vi "Fetch Measurement (Fast Read).vi"(8 "error in (no error)":errorcluster, 10 "Timeout (10000 ms)":u32=10000, 11 "VISA resource name":refnum<visa-resource-name>) -> (0 "error out":errorcluster, 1 "End of Data?":bool, 2 "Measurements":dbl[](array[numeric]) format="%#_24g", 3 "VISA resource name out":refnum<visa-resource-name>)   [LabVIEW 2014, in "Agilent 34401.lvlib"]
doc: "Fetches measurement from the instrument. This VI sends the \"R?\" command to the instrument and is to be used after \"FORM:DATA REAL,64;:FORM:BORD NORM;:INIT;\" has been called. The VI will retrieve and delete the existent data from the instrument's internal buffer. This VI should be called repeatedly until End of Data? is True.\n\n<B>Note:</B>\n\nThis VI is called by <B>Fetch Measurement VI</B> in the following cases:\n(1) Model = 34410/34411 and Math = Off"
uses:
  <instrlib>/Agilent 34401/Agilent 34401.lvlib
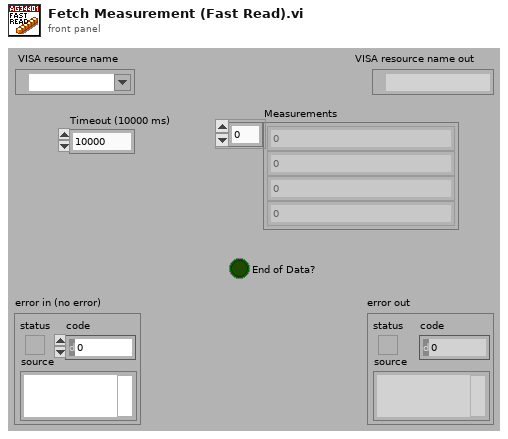
[diagram p1: front panel]
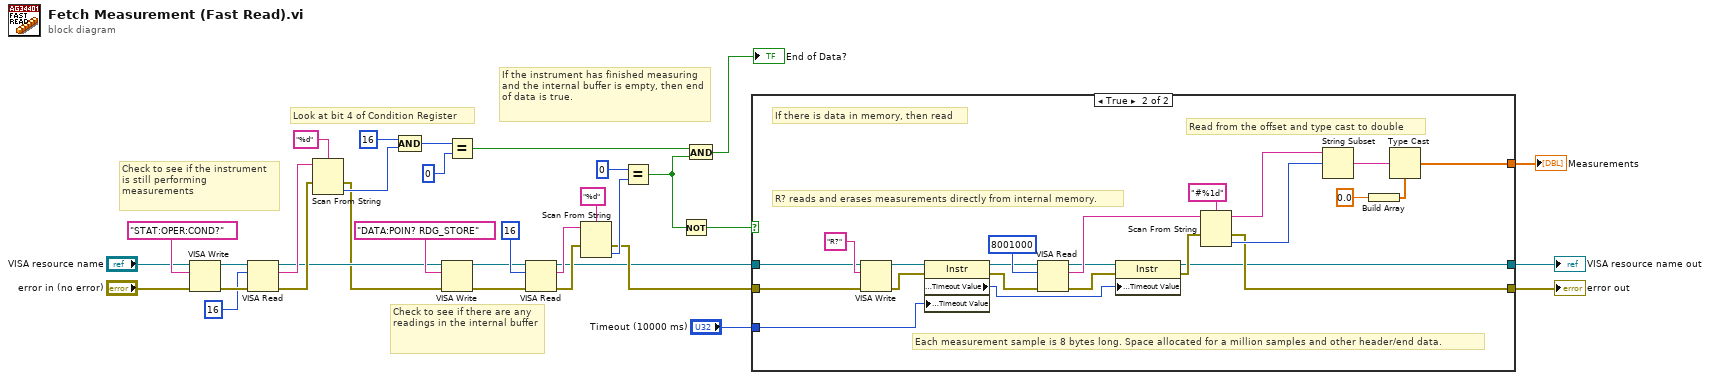
[diagram p0: block diagram]
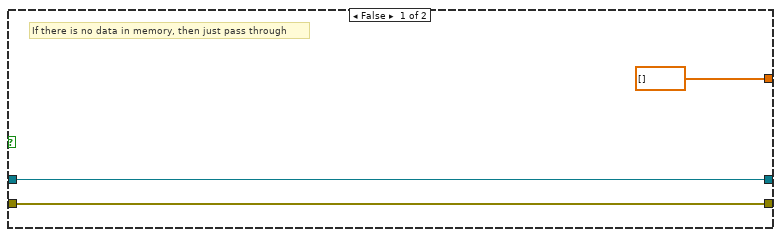
[diagram p2: hidden frame]
diagram:
  # "Look at bit 4 of Condition Register"
  # "If the instrument has finished measuring and the internal buffer is empty, then end of data is true."
  # "Check to see if there are any readings in the internal buffer"
  # "Check to see if the instrument is still performing measurements"
  n1 = VISA Write(VISA resource name="VISA resource name", write buffer="STAT:OPER:COND?", error in (no error)="error in (no error)") -> (VISA resource name out=w27:refnum<visa-resource-name>, error out=w28:errorcluster)  [unwired: 1 out]
  n2 = VISA Read(VISA resource name=w27, byte count=u32 16, error in (no error)=w28) -> (VISA resource name out=w13:refnum<visa-resource-name>, read buffer=w24:string, error out=w15:errorcluster)  [unwired: 1 out]
  n3 = Scan From String(format string="%d", input string=w24, error in=w15) -> (error out=w12:errorcluster, output 1=w21:i32)  [unwired: 2 in, 2 out]
  n4 = Compound Arithmetic op=AND(16 ("value"), w21) -> (w20:i32)
  n5 = VISA Write(VISA resource name=w13, write buffer="DATA:POIN? RDG_STORE", error in (no error)=w12) -> (VISA resource name out=w11:refnum<visa-resource-name>, error out=w33:errorcluster)  [unwired: 1 out]
  n6 = Equal?(x=w20, y=0) -> (x = y?=w14:bool)
  n7 = VISA Read(VISA resource name=w11, byte count=u32 16, error in (no error)=w33) -> (VISA resource name out=w4:refnum<visa-resource-name>, read buffer=w31:string, error out=w16:errorcluster)  [unwired: 1 out]
  n8 = Scan From String(format string="%d", input string=w31, error in=w16) -> (error out=w10:errorcluster, output 1=w23:i32)  [unwired: 2 in, 2 out]
  n9 = Equal?(x=0, y=w23) -> (x = y?=w2:bool)
  n10 = Not(x=w2) -> (.not. x?=w1:bool)
  n11 = And(x=w14, y=w2) -> (x .and. y?=→"End of Data?":bool)
  n12 = case shown="True" w1 {
    tunnel: [dbl[] [] w55] -> w34
    tunnel: w10 -> [w36 w42]
    tunnel: "Timeout (10000 ms)" -> [_ w41]
    tunnel: [w36 w40] -> w6
    tunnel: [w37 w39] -> w5
    tunnel: w4 -> [w37 w38]
    frame False {
      # "If there is no data in memory, then just pass through"
    }
    frame True {
      # "Read from the offset and type cast to double"
      # "If there is data in memory, then read"
      # "Each measurement sample is 8 bytes long. Space allocated for a million samples and other header/end data."
      # "R? reads and erases measurements directly from internal memory."
      n13 = VISA Write(VISA resource name=w38, write buffer="R?", error in (no error)=w42) -> (VISA resource name out=w49:refnum<visa-resource-name>, error out=w48:errorcluster)  [unwired: 1 out]
      n14 = property on="Property Node" class="Instr"(reference=w49, error in=w48, "General Settings:Timeout Value"=w41) -> (reference out=w46:refnum<visa-resource-name>, error out=w47:errorcluster, "General Settings:Timeout Value"=w45:u32)
      n15 = VISA Read(VISA resource name=w46, byte count=u32 8001000, error in (no error)=w47) -> (VISA resource name out=w50:refnum<visa-resource-name>, read buffer=w56:string, error out=w44:errorcluster)  [unwired: 1 out]
      n16 = property on="Property Node" class="Instr"(reference=w50, error in=w44, "General Settings:Timeout Value"=w45) -> (reference out=w39:refnum<visa-resource-name>, error out=w43:errorcluster)
      n17 = Scan From String(format string="#%1d", input string=w56, error in=w43) -> (remaining string=w53:string, error out=w40:errorcluster, output 1=w52:i32)  [unwired: 2 in, 1 out]
      n18 = String Subset(string=w53, offset (0)=w52) -> (substring=w51:string)  [unwired: 1 in]
      n19 = Build Array(0.0) -> (w60:dbl[])
      n20 = Type Cast(type=w60, x=w51) -> (*(type *) &x=w55:dbl[])
    }
  }
  "Measurements" <- w34
  "error out" <- w6
  "VISA resource name out" <- w5
